vi "Get and Decode BTI Activity Error and Command Word.vi"(8 "error in":errorcluster, 10 "message fields":T1 {"data" format="%x"; "extra" format="%x"; "msgopt" format="%04x"; "msgflag" format="%04x"; "bus" items=["BUSA", "BUSB", "BUSNONE"]; "cwd1" format="%04x"; "cwd2" format="%04x"; "swd1" format="%04x"; "swd2" format="%04x"}, 11 "map of messages to value indexes":T3) -> (0 "error out":errorcluster, 2 "message fields out":T1 {"data" format="%x"; "extra" format="%x"; "msgopt" format="%04x"; "msgflag" format="%04x"; "bus" items=["BUSA", "BUSB", "BUSNONE"]; "cwd1" format="%04x"; "cwd2" format="%04x"; "swd1" format="%04x"; "swd2" format="%04x"}, 3 "value":T5, 4 "status error counts":T2, 5 "update values":bool)   [LabVIEW 2023, in "Ballard MIL-STD-1553 Engine Support.lvlib" / "Implementation.lvlib" / "Rx Execution Unit.lvclass"]
uses:
  Rx Execution Unit.lvclass
  Message Map Value.ctl
  Shared/Message Definition.ctl
  Shared/Message Type.ctl
  Shared/Terminal Endpoint.ctl
  Shared/Address.ctl
  Shared/Map of Messages to Value Indexes.ctl
  Shared/Message Map Key.ctl
  Status Error Counts.ctl
  <instrlib>/BTI1553Lib/Public/Controls/1553 Message Fields.ctl
  Rx Execution Unit.lvclass/Rx Execution Unit.ctl
  <instrlib>/BTI1553Lib/BTI1553LV.lvlib
  <vilib>/NI VeriStand/Custom Device Tools/Custom Device Utility Library/Custom Device Utility Library.lvlib
  Shared/Parameter Definition.ctl
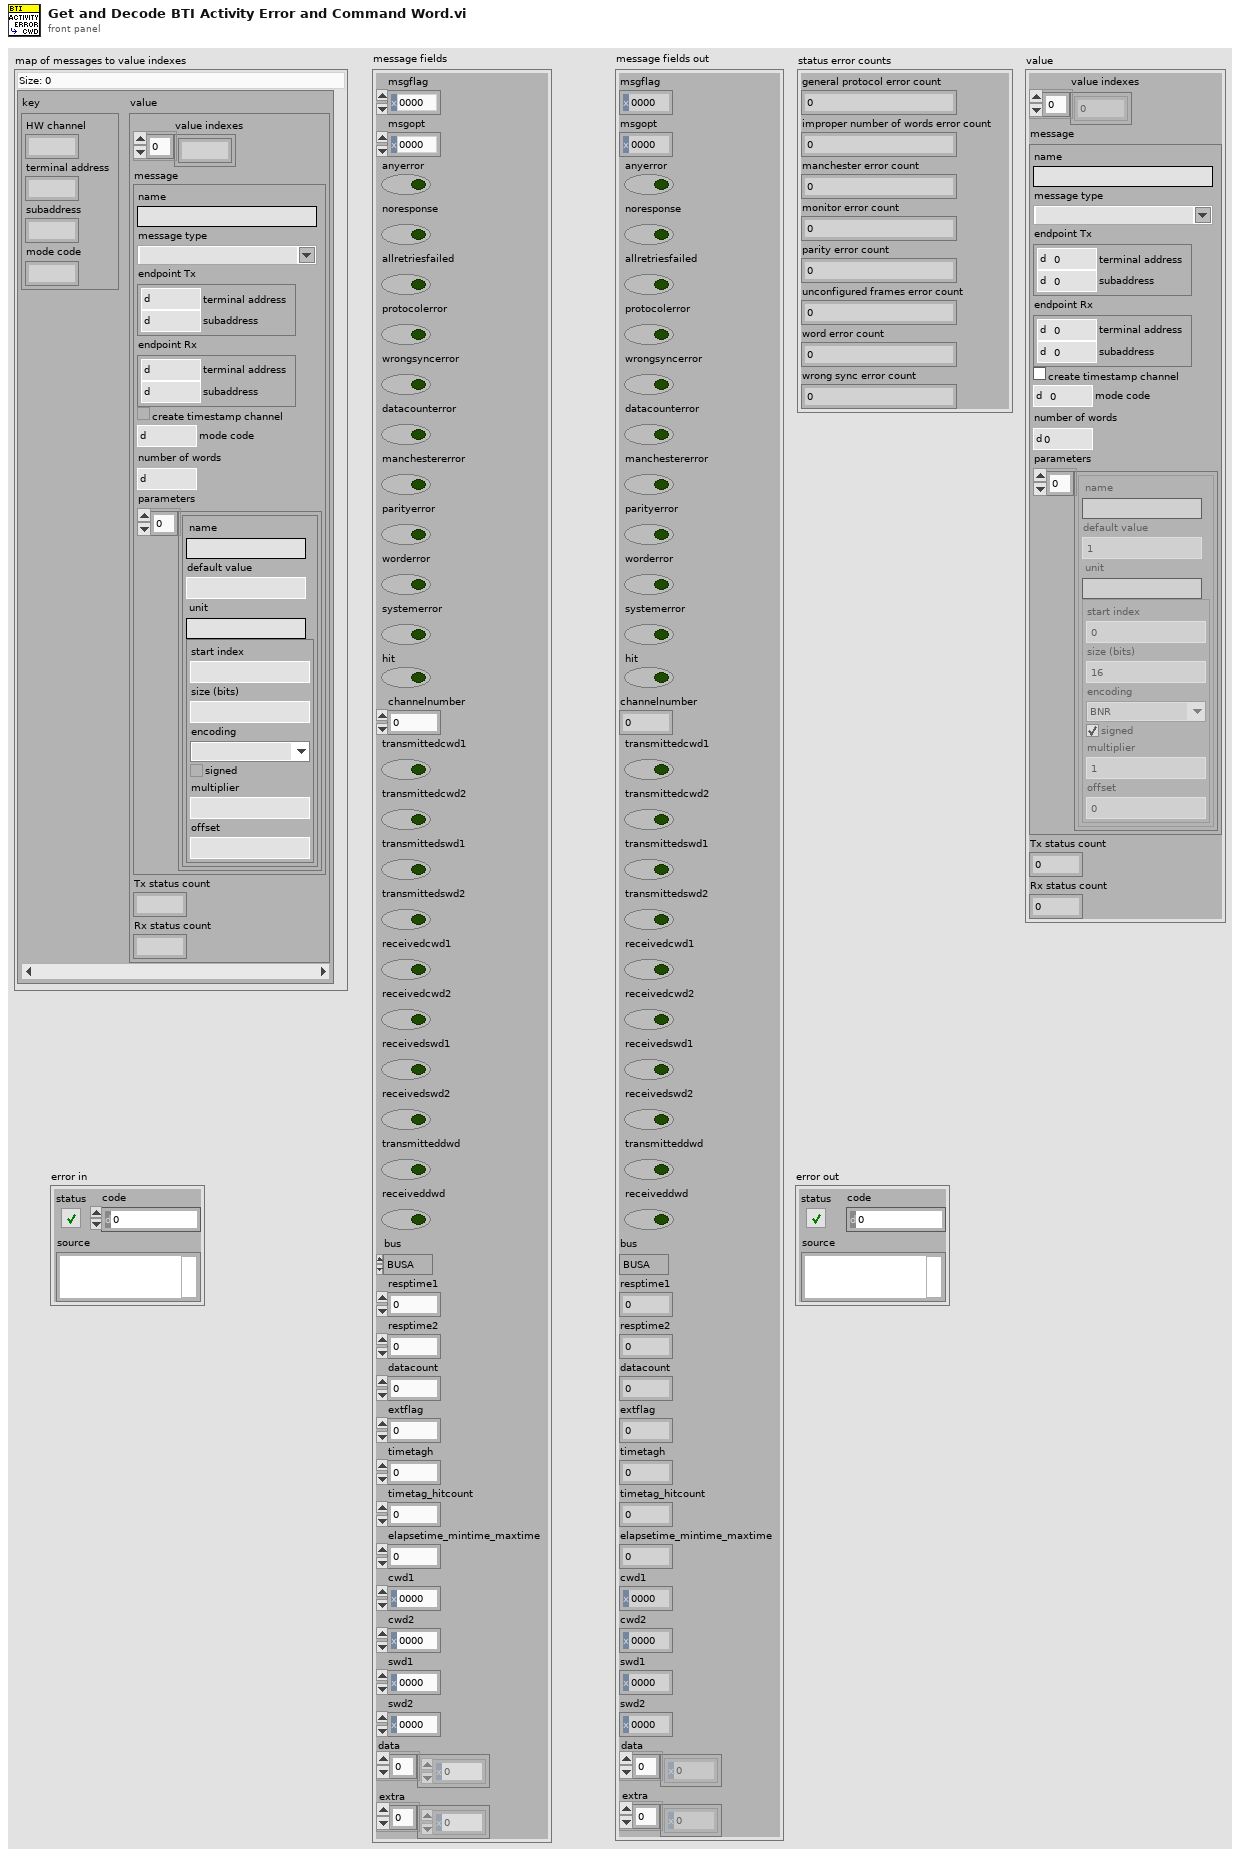
[diagram p1: front panel]
types:
  T1 = typedef "BTI1553LV.lvlib/1553 Message Fields.ctl" = cluster{"msgflag":u16, "msgopt":u16, "anyerror":bool, "noresponse":bool, "allretriesfailed":bool, "protocolerror":bool, "wrongsyncerror":bool, "datacounterror":bool, "manchestererror":bool, "parityerror":bool, "worderror":bool, "systemerror":bool, "hit":bool, "reserved":u8, "channelnumber":i32, "transmittedcwd1":bool, "transmittedcwd2":bool, "transmittedswd1":bool, "transmittedswd2":bool, "receivedcwd1":bool, "receivedcwd2":bool, "receivedswd1":bool, "receivedswd2":bool, "transmitteddwd":bool, "receiveddwd":bool, "reserved":i8, "reserved":i8, "bus":u32, "resptime1":u16, "resptime2":u16, "datacount":u16, "extflag":u16, "timetagh":u32, "timetag_hitcount":u32, "elapsetime_mintime_maxtime":u32, "cwd1":u16, "cwd2":u16, "swd1":u16, "swd2":u16, "data":u16[], "extra":u16[]}
  T2 = typedef "Ballard MIL-STD-1553 Engine Support.lvlib/Implementation.lvlib/Rx Execution Unit.lvclass/Status Error Counts.ctl" = cluster{"general protocol error count":u64, "improper number of words error count":u64, "manchester error count":u64, "monitor error count":u64, "parity error count":u64, "unconfigured frames error count":u64, "word error count":u64, "wrong sync error count":u64}
  T3 = typedef "Map of Messages to Value Indexes.ctl" = map{T4, T5}
  T4 = typedef "Message Map Key.ctl" = cluster{"HW channel":u16, "terminal address":u16, "subaddress":u16, "mode code":u16}
  T5 = typedef "Ballard MIL-STD-1553 Engine Support.lvlib/Implementation.lvlib/Rx Execution Unit.lvclass/Message Map Value.ctl" = cluster{"value indexes":i32[], "message":T6, "Tx status count":i32, "Rx status count":i32}
  T6 = typedef "Message Definition.ctl" = cluster{"name":string, "message type":T7, "endpoint Tx":T8, "endpoint Rx":T8, "create timestamp channel":bool, "mode code":u16, "number of words":u16, "parameters":cluster{"name":string, "default value":dbl, "unit":string, "parameter definition":T10}[]}
  T7 = typedef "Message Type.ctl" = string
  T8 = typedef "Terminal Endpoint.ctl" = cluster{"terminal address":T9, "subaddress":T9}
  T9 = typedef "Address.ctl" = u16
  T10 = typedef "Parameter Definition.ctl" = cluster{"start index":i32, "size (bits)":i32, "encoding":enum16{"BNR", "BCD", "Discrete"}, "signed":bool, "multiplier":dbl, "offset":dbl}
  T11 = cluster{"name":string, "default value":dbl, "unit":string, "parameter definition":T10}[]
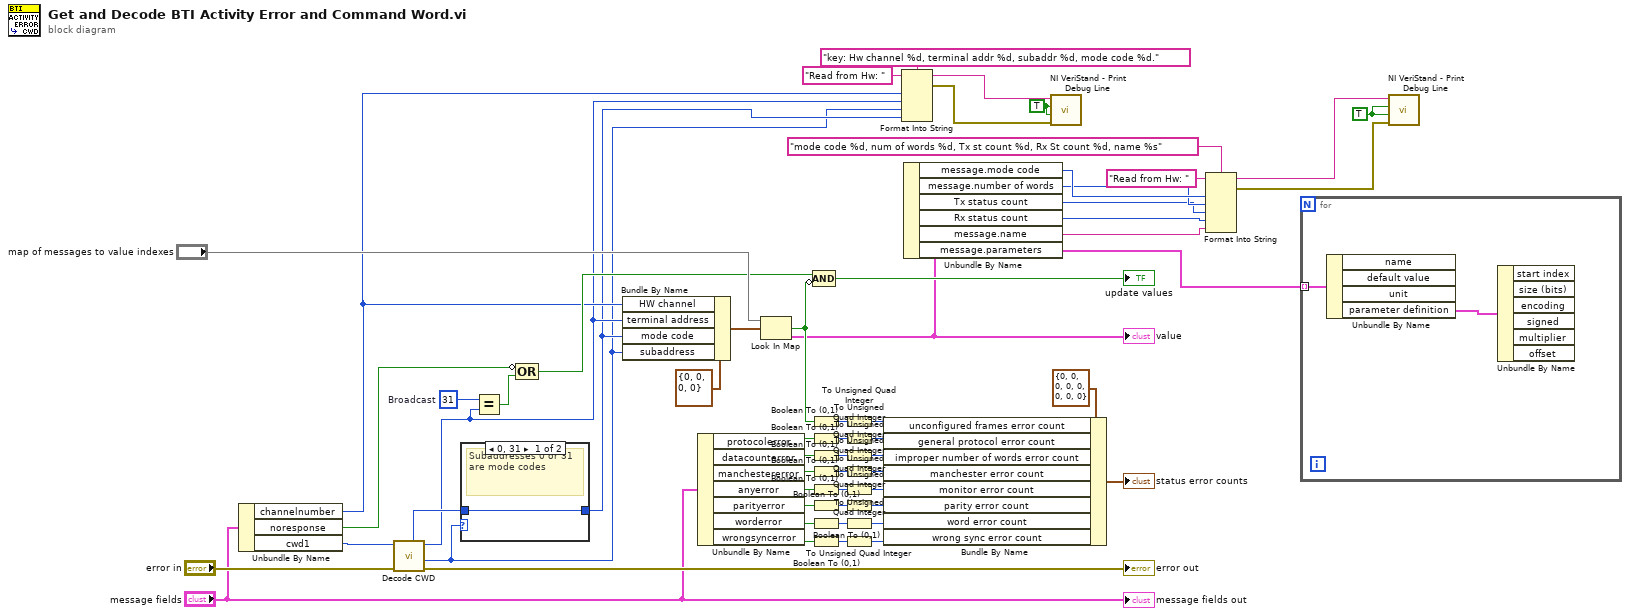
[diagram p0: block diagram]
diagram:
  w5 = TRUE ("Append newline? (T)")
  w19 = TRUE ("Add to log file? (F)")
  w55 = 31  # Broadcast
  n1 = Unbundle By Name("message fields") -> ("channelnumber"=w16:i32, "noresponse"=w24:bool, "cwd1"=w47:u16)
  n2 = call <instrlib>:"Decode CWD.vi"("error in (no error)"="error in", "command word"=w47) -> ("error out"=→"error out":errorcluster, "subaddress out"=w13:i32, "terminal address out"=w15:i32, "word count out"=w56:i32)  [unwired: 5 in, 1 out]
  n3 = case shown="0, 31" w13 {
    tunnel: w56 -> [w61 _]
    tunnel: [w61 _] -> w14
    frame 0, 31 {
      # "Subaddresses 0 or 31 are mode codes"
    }
    frame Default {
    }
  }
  n4 = Equal?(x=w55, y=w15) -> (x = y?=w58:bool)
  n5 = Compound Arithmetic op=OR(invert w24, w58) -> (w48:bool)
  n6 = Bundle By Name(cluster=T4 {"HW channel"=0, "terminal address"=0, "subaddress"=0, "mode code"=0} ("key"), "HW channel"=w16, "terminal address"=w15, "mode code"=w14, "subaddress"=w13) -> (w60:T4)
  n7 = Unbundle By Name("message fields") -> ("protocolerror"=w43:bool, "datacounterror"=w42:bool, "manchestererror"=w41:bool, "anyerror"=w35:bool, "parityerror"=w36:bool, "worderror"=w38:bool, "wrongsyncerror"=w37:bool)
  n8 = Look In Map(map="map of messages to value indexes", key=w60) -> (key not found?=w23:bool, value=w12:T5)  [unwired: 1 in]
  "value" <- w12
  n9 = Boolean To (0,1)(Boolean=w23) -> (0, 1=w52:i16)
  n10 = Boolean To (0,1)(Boolean=w43) -> (0, 1=w45:i16)
  n11 = Boolean To (0,1)(Boolean=w42) -> (0, 1=w40:i16)
  n12 = Boolean To (0,1)(Boolean=w41) -> (0, 1=w34:i16)
  n13 = Boolean To (0,1)(Boolean=w35) -> (0, 1=w33:i16)
  n14 = Boolean To (0,1)(Boolean=w36) -> (0, 1=w32:i16)
  n15 = Boolean To (0,1)(Boolean=w38) -> (0, 1=w31:i16)
  n16 = Boolean To (0,1)(Boolean=w37) -> (0, 1=w30:i16)
  n17 = Compound Arithmetic op=AND(w48, invert w23) -> (→"update values":bool)
  n18 = To Unsigned Quad Integer(1:w52) -> (0:w51:u64)
  n19 = To Unsigned Quad Integer(1:w45) -> (0:w44:u64)
  n20 = To Unsigned Quad Integer(1:w40) -> (0:w39:u64)
  n21 = To Unsigned Quad Integer(1:w34) -> (0:w25:u64)
  n22 = To Unsigned Quad Integer(1:w33) -> (0:w26:u64)
  n23 = To Unsigned Quad Integer(1:w32) -> (0:w27:u64)
  n24 = To Unsigned Quad Integer(1:w31) -> (0:w28:u64)
  n25 = To Unsigned Quad Integer(1:w30) -> (0:w29:u64)
  n26 = Bundle By Name(cluster=T2 {"general protocol error count"=0, "improper number of words error count"=0, "manchester error count"=0, "monitor error count"=0, "parity error count"=0, "unconfigured frames error count"=0, "word error count"=0, "wrong sync error count"=0} ("status error counts"), "unconfigured frames error count"=w51, "general protocol error count"=w44, "improper number of words error count"=w39, "manchester error count"=w25, "monitor error count"=w26, "parity error count"=w27, "word error count"=w28, "wrong sync error count"=w29) -> (→"status error counts":T2)
  n27 = Format Into String(format string="key: Hw channel %d, terminal addr %d, subaddr %d, mode code %d.", initial string="Read from Hw: ", w16, w15, w13, w14) -> (resulting string=w18:string, error out=w17:errorcluster)  [unwired: 1 in]
  n28 = Unbundle By Name(w12) -> ("message.mode code"=w9:u16, "message.number of words"=w8:u16, "Tx status count"=w7:i32, "Rx status count"=w6:i32, "message.name"=w2:string, "message.parameters"=w1:T11)
  n29 = call <vilib>:"NI VeriStand - Print Debug Line.vi"("error in (no error)"=w17, "Append newline? (T)"=w19, "Add to log file? (F)"=w19, "Message"=w18) -> ()  [unwired: 7 in, 1 out]
  n30 = Format Into String(format string="mode code %d, num of words %d, Tx st count %d, Rx St count %d, name %s", initial string="Read from Hw: ", w9, w8, w7, w6, w2) -> (resulting string=w4:string, error out=w3:errorcluster)  [unwired: 1 in]
  n31 = for {
    tunnel: w1 -> [w63] mode=indexing
    n32 = Unbundle By Name(w63) -> ("parameter definition"=w62:T10)  [unwired: 3 out]
    n33 = Unbundle By Name(w62) -> ()  [unwired: 6 out]
  }
  n34 = call <vilib>:"NI VeriStand - Print Debug Line.vi"("error in (no error)"=w3, "Append newline? (T)"=w5, "Add to log file? (F)"=w5, "Message"=w4) -> ()  [unwired: 7 in, 1 out]
  "message fields out" <- "message fields"
